vi "AVI文件读取.vi"() -> ()   [LabVIEW 2018]
uses:
  <vilib>/vision/Avi.llb/IMAQ AVI2 Codec Path.ctl
panel:
  out "error out":errorcluster
  out "Image":T1(plugin-control)
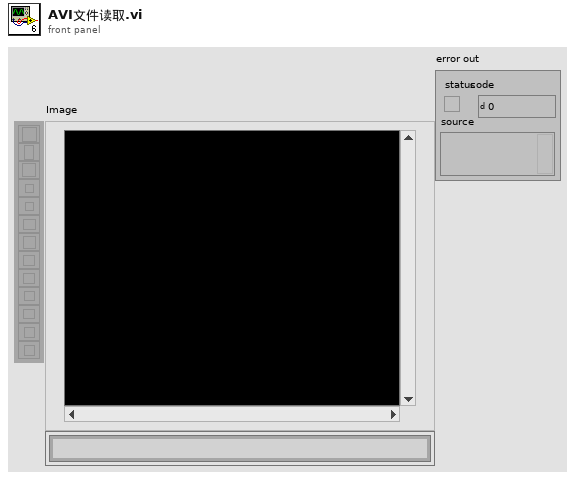
[diagram p1: front panel]
types:
  T1 = typedef "IMAQ Image.ctl" = refnum<image>
  T2 = typedef "IMAQ AVI2 Codec Path.ctl" = u32
  T3 = typedef "IMAQ AVI2 Refnum.ctl" = refnum<k20>
  T4 = typedef "Image Type" = u32
  T5 = cluster{"Width":u32, "Height":u32, "Frames Per Second":u32, "Codec":string, "Has Data":bool}
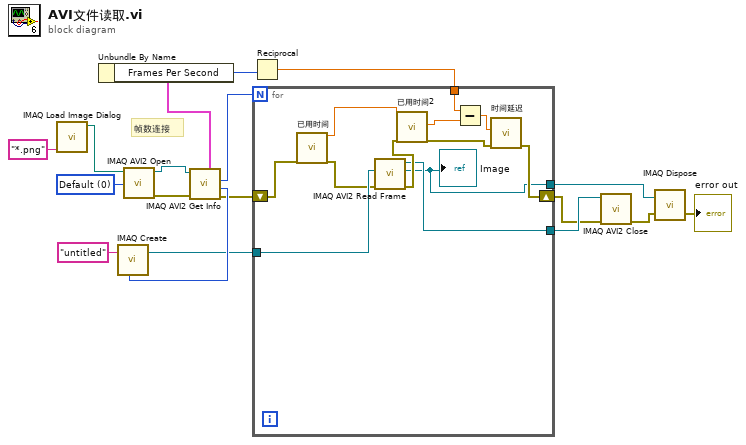
[diagram p0: block diagram]
diagram:
  w16 = T2 0 items=["Default", "System", "Built in Vision"] ("Codec Source")
  # "帧数连接"
  n1 = call "IMAQ Load Image Dialog"("Pattern"="*.png") -> ("Path"=w17:path)  [unwired: 8 in, 2 out]
  n2 = call "IMAQ AVI2 Open"("Codec Source"=w16, "AVI File Path"=w17) -> ("error out"=w9:errorcluster, "AVI Refnum"=w15:T3)  [unwired: 8 in]
  n3 = call "IMAQ AVI2 Get Info"("error in (no error)"=w9, "AVI Refnum"=w15) -> ("error out"=w10:errorcluster, "Image Type"=w12:T4, "Number of Frames"=w14:u32, "Frame Data"=w8:T5)  [unwired: 5 in, 1 out]
  n4 = Unbundle By Name(w8) -> ("Frames Per Second"=w7:u32)
  n5 = call "IMAQ Create"("Image Name"="untitled", "Image Type"=w12) -> ("New Image"=w11:T1)  [unwired: 3 in, 1 out]
  n6 = Reciprocal(x=w7) -> (1/x=w6:dbl)
  n7 = for {
    N: w14 -> [_]
    tunnel: w11 -> [w30]
    shift-right: [w21] -> w4
    shift-left: w10 -> [w29]
    tunnel: w6 -> [w24]
    tunnel: [w20] -> w5
    tunnel: [w19] -> w3
    n8 = call "已用时间"("error in (no error)"=w29) -> ("Present (s)"=w26:dbl, "error out"=w28:errorcluster)  [unwired: 11 in, 6 out]
    n9 = call "IMAQ AVI2 Read Frame"("error in (no error)"=w28, "Image"=w30) -> ("error out"=w27:errorcluster, "Image Out"=w19:T1, "AVI Refnum (duplicate)"=w20:T3)  [unwired: 7 in]
    "Image" <- w19
    n10 = call "已用时间2"("error in (no error)"=w27, "Set Start Time (s)"=w26) -> ("Elapsed Time (s)"=w25:dbl, "error out"=w22:errorcluster)  [unwired: 10 in, 6 out]
    n11 = Subtract(x=w24, y=w25) -> (x-y=w23:dbl)
    n12 = call "时间延迟"("error in (no error)"=w22, "Delay Time (s)"=w23) -> ("error out"=w21:errorcluster)  [unwired: 9 in]
  }
  n13 = call "IMAQ AVI2 Close"("error in (no error)"=w4, "AVI Refnum"=w5) -> ("error out"=w2:errorcluster)  [unwired: 9 in]
  n14 = call "IMAQ Dispose"("Image"=w3, "error in (no error)"=w2) -> ("error out"=→"error out":errorcluster)  [unwired: 4 in]
